vi "modbusRxTelemetryUpdateLoop.vi"(11 "Modbus Port Settings":T1={"Tx Port"="ModbusPort1Tx", "Tx Data FIFO"="txModbusPort1FIFO", "Tx Internal FIFO"="txModbusPort1InternalFIFO", "Tx Telemetry FIFO"="txModbusPort1TelemetryFIFO", "Rx Port"="ModbusPort1Rx", "Rx Data FIFO"="rxModbusPort1FIFO", "Rx Telemetry FIFO"="txModbusPort1TelemetryFIFO", "Base Telemetry Address"=0, "Wait For Rx Frame Register"="WaitForRxFrame", "IRQ Address"=0, "Trigger IRQ Register"="TriggerPort1IRQ", "Trigger IRQ Response Register"="TriggerPort1IRQ"}) -> ()   [LabVIEW 2015]
uses:
  DataTypes/ModbusPortSettings.ctl
  <vilib>/rvi/Emulation/niFpgaGetClockAttributes.vi
  <vilib>/rvi/Emulation/niFpgaSctlEmulationGetInTimedLoop.vi
  <vilib>/rvi/Emulation/niFpgaEmulationReportErrorSimple.vi
  <vilib>/rvi/Emulation/niFpgaEmulationIsFPGAContextNoSignature.vi
  <vilib>/rvi/DataTransferAndStorage/Container/Common/niFpgaContainerGetUniqueNameForEmu.vi
  <vilib>/rvi/Memory/Memory_Emulation/niFpgaMemoryEmulationCacheClearOnFirstRun.vi
  <vilib>/rvi/Memory/Memory_Emulation/nirvimemoryEmulationManagerCache_MakeExclusive.vi
  <vilib>/rvi/Memory/Memory_Emulation/niFpgaMemoryEmulationValidateCache.vi
  <vilib>/rvi/Memory/Memory_Emulation/nirvimemoryEmulationManagerCache_InsertValue.vi
  <vilib>/Utility/error.llb/Clear Errors.vi
  <vilib>/rvi/Memory/Memory_Emulation/nirvimemoryEmulationManagerCache_ReleaseExclusive.vi
  <vilib>/rvi/Memory/Memory_Emulation/nirvimemoryEmulationManagerCache_GetValue.vi
  <vilib>/rvi/Memory/Memory_Emulation/nirvimemoryEmulationManagerCache_SetValue.vi
  <vilib>/rvi/Emulation/niFpgaProcessEmulError.vi
  <vilib>/rvi/DataTransferAndStorage/Container/Common/niFpgaContainerExecOnDevCompGetState.vi
  <vilib>/rvi/errors/niFpgaSetErrorForExecOnDevCompSimple.vi
  <vilib>/rvi/eio/common/nirviEmuReportErrorAndStop.vi
  <vilib>/rvi/FIFO/Fifo_Resource/nirvififoEmulationSetSize.vi
  <vilib>/rvi/FIFO/Fifo_Resource/nirviFifoEmulationQueueMgr.vi
  <instcachedir>/0/nirviFifoEmulationQueueMgr_E5CAEC123FF24DC58D834DCA3CDAA9B5.lvgen/nirviFifoEmulationQueueMgr_E5CAEC123FF24DC58D834DCA3CDAA9B5_008.vi
  <vilib>/rvi/FIFO/Fifo_Resource/nirvififoEmulationDetermineInputValidOut.vi
  <vilib>/rvi/FIFO/Fifo_Resource/nirvififoEmulationCreateLock.vi
  <vilib>/rvi/FIFO/Fifo_Resource/nirvififoEmulationObtainLock.vi
  <vilib>/rvi/FIFO/Fifo_Resource/nirvififoEmulationReleaseLock.vi
  <vilib>/rvi/occurrence/nirviWaitOnOccurrenceBase.vi
  <vilib>/rvi/errors/nirviReportUnexpectedCaseInternalError.vi
  <vilib>/rvi/errors/nirviReportUnexpectedCaseInternalError (U32).vi
  <vilib>/rvi/interface/RandomDataEmulation/niFpgaRandomDataHandleErrors.vi
  <vilib>/rvi/Emulation/niFpgaCriticalErrorInLSC.vi
  <vilib>/rvi/DataTransferAndStorage/Container/XNode/niFpgaContainer.xnode
  <vilib>/rvi/DataTransferAndStorage/Register/Emulation/niFpgaRegisterEmulation.vi
  <vilib>/rvi/FIFO/Fifo_Resource/niFpgaFifoEmulationRefIn.vi
  <vilib>/rvi/FIFO/Fifo_Resource/nirvififoEmulationWrite.vi
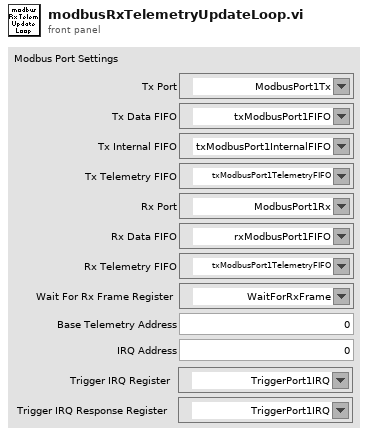
[diagram p1: front panel]
types:
  T1 = typedef "ModbusPortSettings.ctl" = cluster{"Tx Port":refnum<k21>, "Tx Data FIFO":refnum<k21>, "Tx Internal FIFO":refnum<k21>, "Tx Telemetry FIFO":refnum<k21>, "Rx Port":refnum<k21>, "Rx Data FIFO":refnum<k21>, "Rx Telemetry FIFO":refnum<k21>, "Base Telemetry Address":u32, "Wait For Rx Frame Register":refnum<k21>, "IRQ Address":u8, "Trigger IRQ Register":refnum<k21>, "Trigger IRQ Response Register":refnum<k21>}
  T2 = cluster{"Address":u32, "Telemetry Update Mode":enum8{"NOP", "Set", "Add", "Subtract", "Or"}, "Data":u32}
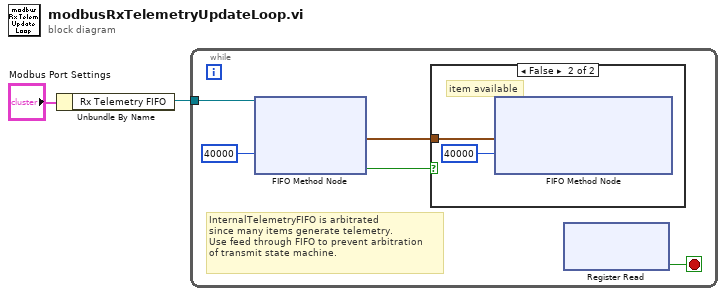
[diagram p0: block diagram]
diagram:
  n1 = Unbundle By Name("Modbus Port Settings") -> ("Rx Telemetry FIFO"=w1:refnum<k21>)
  n2 = while {
    tunnel: w1 -> [w5]
    stop <- w7 stop-if-true
    # "InternalTelemetryFIFO is arbitrated\nsince many items generate telemetry.\nUse feed through FIFO to prevent arbitration\nof transmit state machine."
    n3 = xnode ("FIFO Method Node")("Timeout"=40000, "FIFO In"=w5) -> ("Element"=w6:T2, "Timed Out?"=w3:bool)  [unwired: 1 out]
    n4 = case shown="False" w3 {
      tunnel: w6 -> [_ w8]
      frame True {
        # "no item available"
      }
      frame False {
        # "item available"
        n5 = xnode ("FIFO Method Node")("Element"=w8, "Timeout"=40000) -> ()  [unwired: 1 in, 2 out]
      }
    }
    n6 = xnode ("Register Read")() -> ("Data"=w7:bool)  [unwired: 1 in, 1 out]
  }
